vi "Exe.vi"(0 "reference in":refnum<class "Context.lvclass">, 5 "error in (no error)":errorcluster) -> (14 "reference out":refnum<class "Context.lvclass">, 15 "result":dbl, 19 "error out":errorcluster)   [LabVIEW 2013, in "Context.lvclass"]
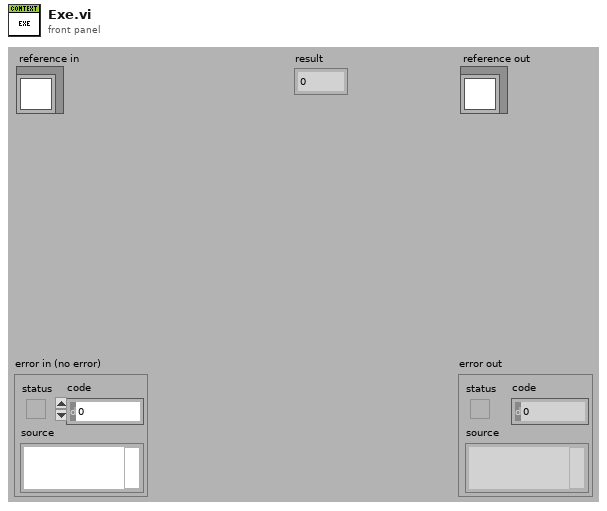
[diagram p1: front panel]
types:
  T1 = typedef "Context.lvclass/ObjectAttributes.ctl" = cluster{"Operation.lvclass":refnum<class "Operation.lvclass">}
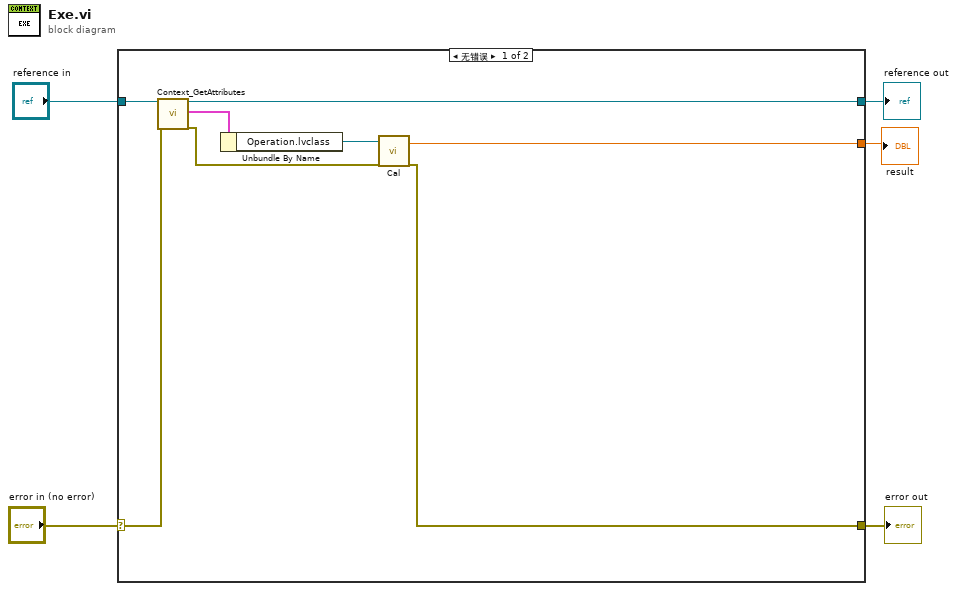
[diagram p0: block diagram]
diagram:
  n1 = case shown="无错误" "error in (no error)" {
    selector: "error in (no error)" -> [w13 w15]
    tunnel: [w7 w15] -> w4
    tunnel: [w12 w14] -> w2
    tunnel: "reference in" -> [w10 w14]
    tunnel: [w6 _] -> w1
    frame No Error {
      n2 = call "Context_GetAttributes.vi"("reference in"=w10, "error in (no error)"=w13) -> ("reference out"=w12:refnum<class "Context.lvclass">, "attributes"=w11:T1, "error out"=w8:errorcluster)  [unwired: 14 in, 1 out]
      n3 = Unbundle By Name(w11) -> ("Operation.lvclass"=w9:refnum<class "Operation.lvclass">)
      n4 = call-dynamic "Cal.vi"("reference in"=w9, "error in (no error)"=w8) -> ("result"=w6:dbl, "error out"=w7:errorcluster)  [unwired: 15 in, 1 out]
    }
    frame Error {
    }
  }
  "error out" <- w4
  "reference out" <- w2
  "result" <- w1
